vi "IndexToArray.vi"(8 "error in":errorcluster caption="错误输入", 10 "Extract":T1(ring), 11 "Setup":T2) -> (0 "error out":errorcluster caption="错误输出", 3 "Value":string[][](array[string]))   [LabVIEW 2013]
uses:
  SetupCtl.ctl
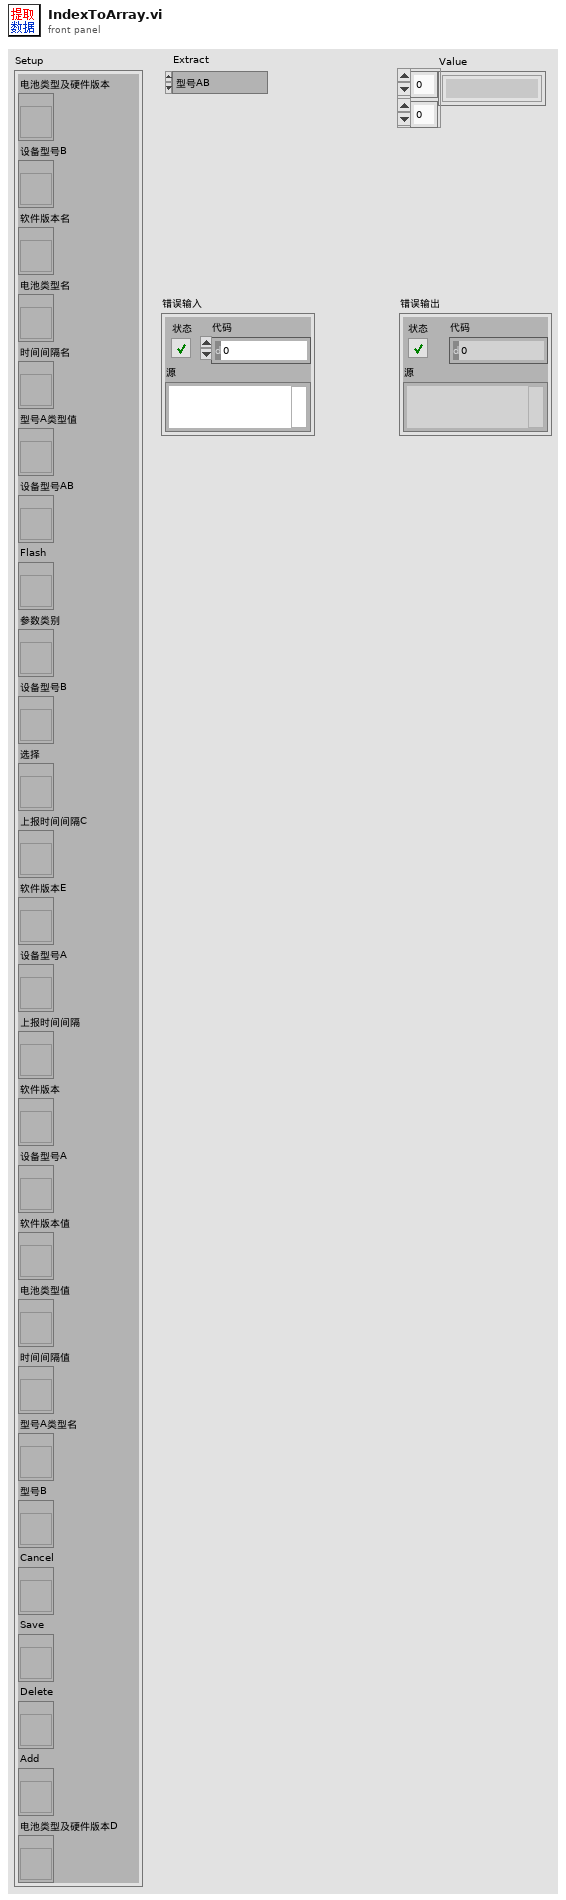
[diagram p1: front panel]
types:
  T1 = enum16{"型号AB", "型号A", "型号B", "上报时间间隔", "电池类型", "软件版本"}
  T2 = typedef "SetupCtl.ctl" = cluster{"电池类型及硬件版本":refnum<vi>, "设备型号B":refnum<vi>, "软件版本名":refnum<vi>, "电池类型名":refnum<vi>, "时间间隔名":refnum<vi>, "型号A类型值":refnum<vi>, "设备型号AB":refnum<vi>, "Flash":refnum<vi>, "参数类别":refnum<vi>, "设备型号B":refnum<vi>, "选择":refnum<vi>, "上报时间间隔C":refnum<vi>, "软件版本E":refnum<vi>, "设备型号A":refnum<vi>, "上报时间间隔":refnum<vi>, "软件版本":refnum<vi>, "设备型号A":refnum<vi>, "软件版本值":refnum<vi>, "电池类型值":refnum<vi>, "时间间隔值":refnum<vi>, "型号A类型名":refnum<vi>, "型号B":refnum<vi>, "Cancel":refnum<vi>, "Save":refnum<vi>, "Delete":refnum<vi>, "Add":refnum<vi>, "电池类型及硬件版本D":refnum<vi>}
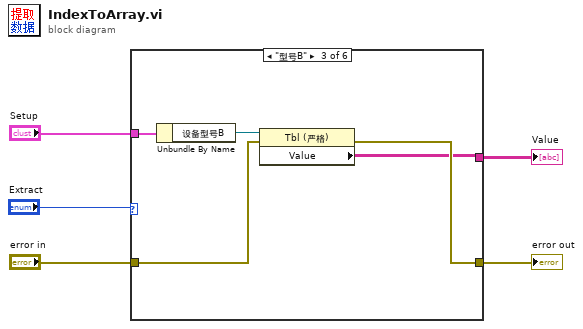
[diagram p0: block diagram]
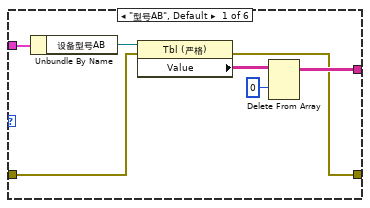
[diagram p2: hidden frame]
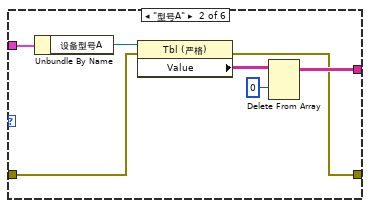
[diagram p3: hidden frame]
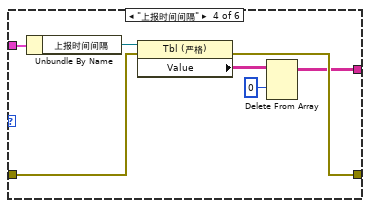
[diagram p4: hidden frame]
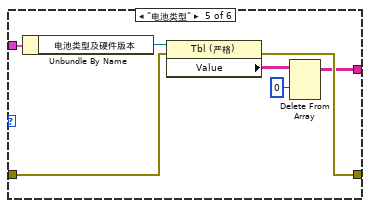
[diagram p5: hidden frame]
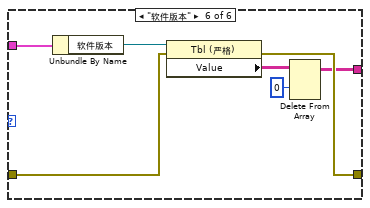
[diagram p6: hidden frame]
diagram:
  n1 = case shown="\"型号B\"" "Extract" {
    tunnel: "Setup" -> [w12 w19 w24 w31 w38 w45]
    tunnel: [w8 w15 w20 w25 w32 w39] -> w3
    tunnel: "error in" -> [w7 w14 w22 w29 w36 w43]
    tunnel: [w6 w13 w21 w28 w35 w42] -> w1
    frame "型号AB", Default {
      n2 = Unbundle By Name(w12) -> ("设备型号AB"=w11:refnum<vi>)
      n3 = property class="Tbl (严格)"(reference=w11, error in=w7) -> (error out=w6:errorcluster, "Value"=w10:string[][])  [unwired: 1 out]
      n4 = Delete From Array(array=w10, index (row)=0 ("索引 (行)")) -> (array with subset deleted=w8:string[][])  [unwired: 2 in, 1 out]
    }
    frame "型号A" {
      n5 = Unbundle By Name(w19) -> ("设备型号A"=w18:refnum<vi>)
      n6 = property class="Tbl (严格)"(reference=w18, error in=w14) -> (error out=w13:errorcluster, "Value"=w17:string[][])  [unwired: 1 out]
      n7 = Delete From Array(array=w17, index (row)=0 ("索引 (行)")) -> (array with subset deleted=w15:string[][])  [unwired: 2 in, 1 out]
    }
    frame "型号B" {
      n8 = Unbundle By Name(w24) -> ("设备型号B"=w23:refnum<vi>)
      n9 = property class="Tbl (严格)"(reference=w23, error in=w22) -> (error out=w21:errorcluster, "Value"=w20:string[][])  [unwired: 1 out]
    }
    frame "上报时间间隔" {
      n10 = Unbundle By Name(w31) -> ("上报时间间隔"=w30:refnum<vi>)
      n11 = property class="Tbl (严格)"(reference=w30, error in=w29) -> (error out=w28:errorcluster, "Value"=w26:string[][])  [unwired: 1 out]
      n12 = Delete From Array(array=w26, index (row)=0 ("索引 (行)")) -> (array with subset deleted=w25:string[][])  [unwired: 2 in, 1 out]
    }
    frame "电池类型" {
      n13 = Unbundle By Name(w38) -> ("电池类型及硬件版本"=w37:refnum<vi>)
      n14 = property class="Tbl (严格)"(reference=w37, error in=w36) -> (error out=w35:errorcluster, "Value"=w33:string[][])  [unwired: 1 out]
      n15 = Delete From Array(array=w33, index (row)=0 ("索引 (行)")) -> (array with subset deleted=w32:string[][])  [unwired: 2 in, 1 out]
    }
    frame "软件版本" {
      n16 = Unbundle By Name(w45) -> ("软件版本"=w44:refnum<vi>)
      n17 = property class="Tbl (严格)"(reference=w44, error in=w43) -> (error out=w42:errorcluster, "Value"=w40:string[][])  [unwired: 1 out]
      n18 = Delete From Array(array=w40, index (row)=0 ("索引 (行)")) -> (array with subset deleted=w39:string[][])  [unwired: 2 in, 1 out]
    }
  }
  "error out" <- w1
  "Value" <- w3
